vi "FTW-Linker-LVFileStaticLinks.vi"(0 "LabVIEW Files":path[](array[path]), 5 "Recursive":bool=TRUE, 11 "error in":errorcluster) -> (4 "LinkerInfo":T1[](array[typedef]) {"iState" format="%08x"; "iStyle" format="%08x"; "wStyle" format="%08x"; "buttons" format="%08x"; "viflags" format="%08x"; "viflags2" format="%08x"}, 15 "error out":errorcluster)   [LabVIEW 2014]
uses:
  FTW-Linker-LinkerInfoStructure.ctl
  FTW-Linker-LabVIEWFiletype.ctl
panel:
  # "Inputs"
  # "Outputs"
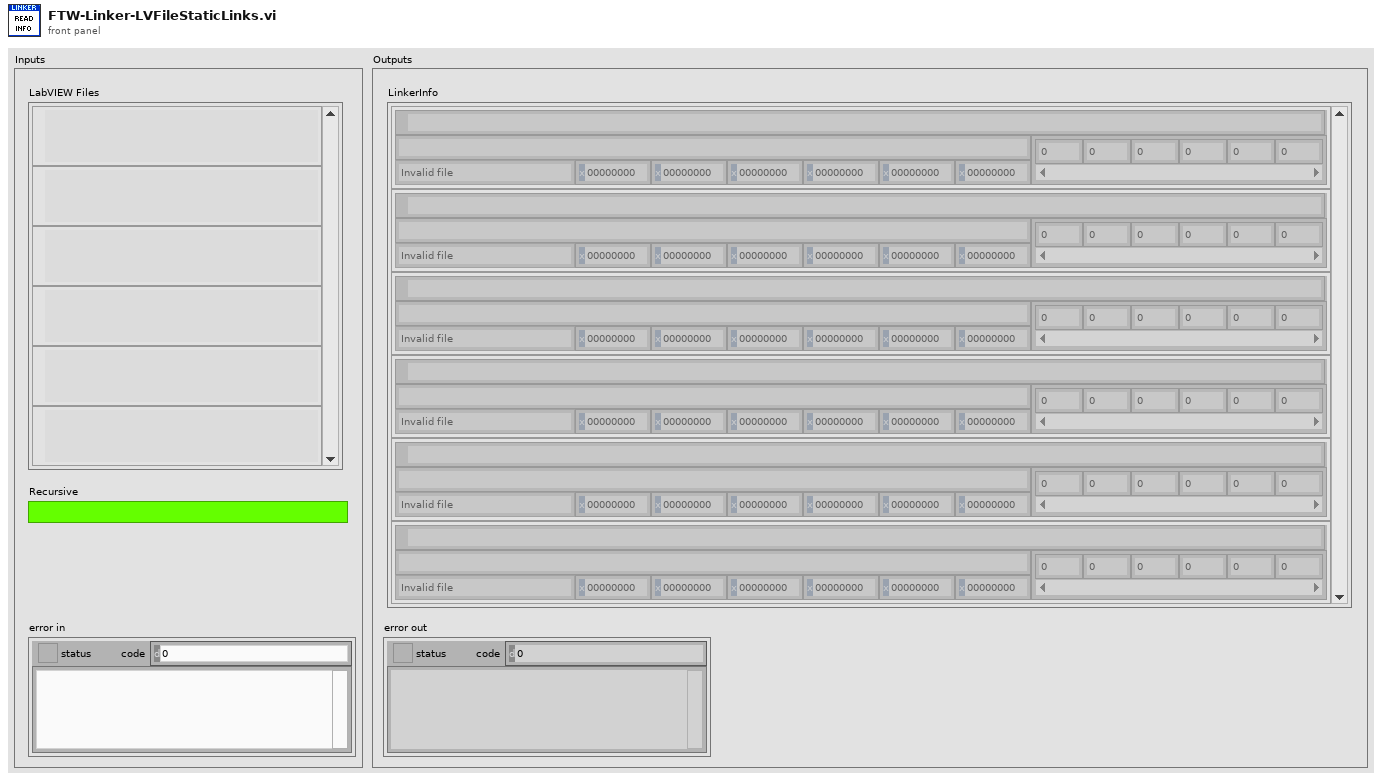
[diagram p1: front panel]
types:
  T1 = typedef "FTW-Linker-LinkerInfoStructure.ctl" = cluster{"path":path, "delimited name":string, "Filetype":T2, "iState":u32, "iStyle":u16, "wStyle":u16, "buttons":u16, "viflags":u32, "viflags2":u32, "links":u32[]}
  T2 = typedef "FTW-Linker-LabVIEWFiletype.ctl" = enum32{"Invalid file", "Unknown type", "VI", "Control", "PolyVI", "Project", "Library", "LVClass", "XControl", "XNode", "Shared Library", "dotNET assembly", "ActiveX interface", "CIN", "Run-time menu", "Palette menu", "Help file", "LLB", "XNode Edit Dependency", "LVClass Private Data", "Statechart", "MathScript .m file", "Ladder Diagram", "Packed Project Lib", "XNode Build Dependency"}
  T3 = typedef "NI_FileType.lvlib/LVFileType.ctl" = enum32{"Invalid file", "Unknown type", "Instrument", "Control", "Polymorphic VI", "Project", "Library", "LVClass", "XControl", "XNode", "Shared library", ".NET assembly", "ActiveX interface", "CIN", "Run-time menu", "Palette menu", "Help file", "LLB", "XNode Edit Dependency", "Class Private Data Control", "Statechart", "MathScript .m file", "Ladder Diagram", "LVLibp", "XNode Build Dependency"}
  T4 = cluster{"path":path, "delimited name":string, "type":T3, "iState":u32, "iStyle":u16, "wStyle":u16, "buttons":u16, "viflags":u32, "viflags2":u32, "links":u32[]}[]
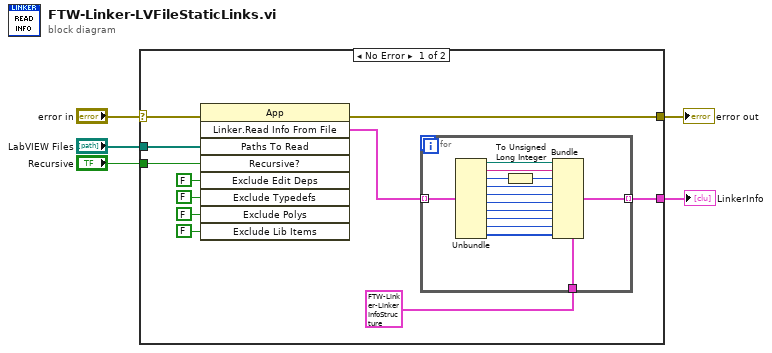
[diagram p0: block diagram]
diagram:
  n1 = case shown="No Error" "error in" {
    selector: "error in" -> [w10 w31]
    tunnel: [w16 w31] -> w5
    tunnel: "Recursive" -> [w15 _]
    tunnel: [w13 _] -> w3
    tunnel: "LabVIEW Files" -> [w11 _]
    frame No Error {
      n2 = invoke class="App" method="Linker.Read Info From File"(error in=w10, "Paths To Read"=w11, "Recursive?"=w15, "Exclude Edit Deps"=FALSE ("Exclude Edit Time Dependencies"), "Exclude Typedefs"=FALSE, "Exclude Polys"=FALSE ("Exclude Poly VIs"), "Exclude Lib Items"=FALSE ("Exclude Unused Library Items")) -> (error out=w16:errorcluster, "Linker.Read Info From File"=w14:T4)  [unwired: 2 in, 7 out]
      n3 = for {
        tunnel: w14 -> [w30] mode=indexing
        tunnel: [w28] -> w13 mode=indexing
        tunnel: T1 {"path"=path "", "delimited name"="", "Filetype"=enum."Invalid file", "iState"=0, "iStyle"=0, "wStyle"=0, "buttons"=0, "viflags"=0, "viflags2"=0, "links"=[]} ("Linker Info") -> [w29]
        n4 = Unbundle(w30) -> ("path"=w27:path, "delimited name"=w26:string, "type"=w18:T3, "iState"=w25:u32, "iStyle"=w24:u16, "wStyle"=w23:u16, "buttons"=w22:u16, "viflags"=w21:u32, "viflags2"=w20:u32, "links"=w19:u32[])
        n5 = To Unsigned Long Integer(number=w18) -> (unsigned 32bit integer=w17:u32)
        n6 = Bundle(cluster=w29, "path"=w27, "delimited name"=w26, "Filetype"=w17, "iState"=w25, "iStyle"=w24, "wStyle"=w23, "buttons"=w22, "viflags"=w21, "viflags2"=w20, "links"=w19) -> (w28:T1)
      }
    }
    frame Error {
    }
  }
  "error out" <- w5
  "LinkerInfo" <- w3
